vi "createInboundChannel.vi"(8 "error in (no error)":errorcluster, 11 "Connection.LocalQueue in":refnum<class "Connection.LocalQueue.lvclass">) -> (0 "error out":errorcluster, 2 "Authorization":T1, 3 "Connection.LocalQueue out":refnum<class "Connection.LocalQueue.lvclass">)   [LabVIEW 2013, in "Connection.Queue_GOSPL.lvlib" / "Connection.LocalQueue.lvclass"]
uses:
  Connection.LocalQueue.lvclass
  Connection/auth -- cluster.ctl
  Connection/Connection.lvclass/Connection.ctl
  Connection/Connection.lvclass
  Connection.LocalQueue.lvclass/Connection.LocalQueue.ctl
  <vilib>/LabVIEW Open Source Project/Unicity/RandomStringGenerator/RandomStringGenerator.lvclass
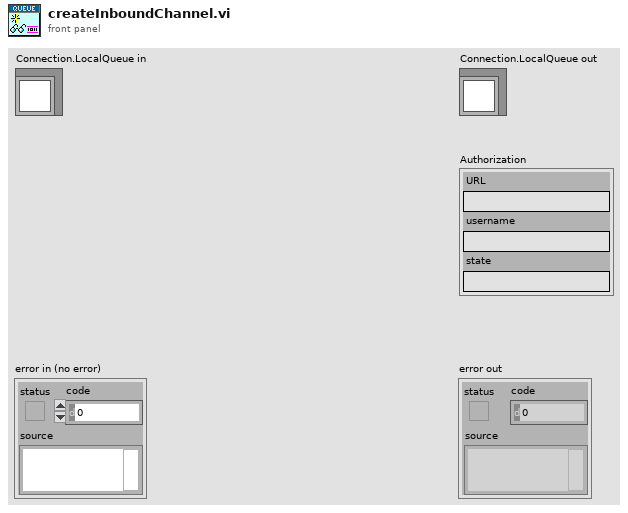
[diagram p1: front panel]
types:
  T1 = typedef "Connection_GOSPL.lvlib/Connection.lvclass/auth -- cluster.ctl" = cluster{"URL":string, "username":string, "state":string}
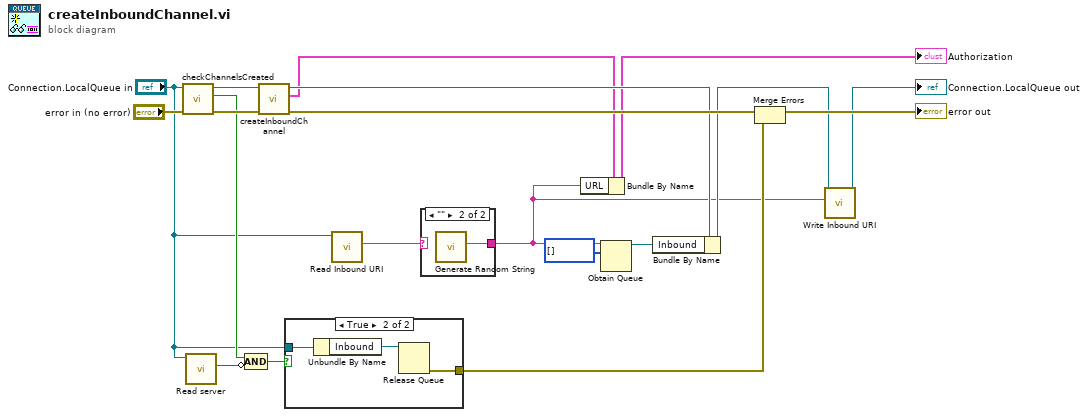
[diagram p0: block diagram]
diagram:
  n1 = call-dynamic "checkChannelsCreated.vi"("error in (no error)"="error in (no error)", "Connection.LocalQueue in"="Connection.LocalQueue in") -> ("error out"=w18:errorcluster, "inbound created"=w12:bool, "Connection.LocalQueue out"=w17:refnum<class "Connection.LocalQueue.lvclass">)  [unwired: 6 in, 1 out]
  n2 = call "Read server.vi"("Connection in"="Connection.LocalQueue in") -> ("server"=w7:bool)  [unwired: 9 in, 1 out]
  n3 = Compound Arithmetic op=AND(w12, invert w7) -> (w11:bool)
  n4 = call-parent "createInboundChannel.vi"("error in (no error)"=w18, "Connection in"=w17) -> ("error out"=w19:errorcluster, "Authorization"=w4:T1, "Connection out"=w16:refnum<class "Connection.LocalQueue.lvclass">)  [unwired: 7 in]
  n5 = case shown="True" w11 {
    tunnel: "Connection.LocalQueue in" -> [_ w21]
    tunnel: [_ w20] -> w10
    frame False {
    }
    frame True {
      n6 = Unbundle By Name(w21) -> ("Inbound"=w22:refnum<queue>)
      n7 = Release Queue(queue=w22) -> (error out=w20:errorcluster)  [unwired: 2 in, 2 out]
    }
  }
  n8 = call "Read Inbound URI.vi"("Connection in"="Connection.LocalQueue in") -> ("Inbound URI"=w2:string)  [unwired: 9 in, 1 out]
  n9 = case shown="\"\"" w2 {
    selector: w2 -> [w23 _]
    tunnel: [w23 w24] -> w5
    frame Default {
    }
    frame "" {
      n10 = call <vilib>:"Generate Random String.vi"() -> ("Random String"=w24:string)  [unwired: 11 in]
    }
  }
  n11 = Bundle By Name(cluster=w4, "URL"=w5) -> (→"Authorization":T1)
  n12 = Obtain Queue(name (unnamed)=w5, element data type=u8[] [] ("Bytes Array")) -> (queue out=w13:refnum<queue>)  [unwired: 3 in, 2 out]
  n13 = Bundle By Name(cluster=w16, "Inbound"=w13) -> (w9:refnum<class "Connection.LocalQueue.lvclass">)
  n14 = Merge Errors(w19, w10) -> (→"error out":errorcluster)
  n15 = call "Write Inbound URI.vi"("Inbound URI"=w5, "Connection in"=w9) -> ("Connection out"=→"Connection.LocalQueue out":refnum<class "Connection.LocalQueue.lvclass">)  [unwired: 9 in]
